vi "network-get_adapters.vi"(8 "error in (no error)":errorcluster) -> (0 "error out":errorcluster, 3 "adapter []":T1[](array[typedef]))   [LabVIEW 2015, in "lv-bin-windows.lvlib" / "v1.lvlib"]
uses:
  v1.lvlib
  _controls/adapter.ctl
  <userlib>/antonio-alexander/lv-bin/lv-bin/public/api/v1/v1.lvlib
panel:
  out "standard output":string
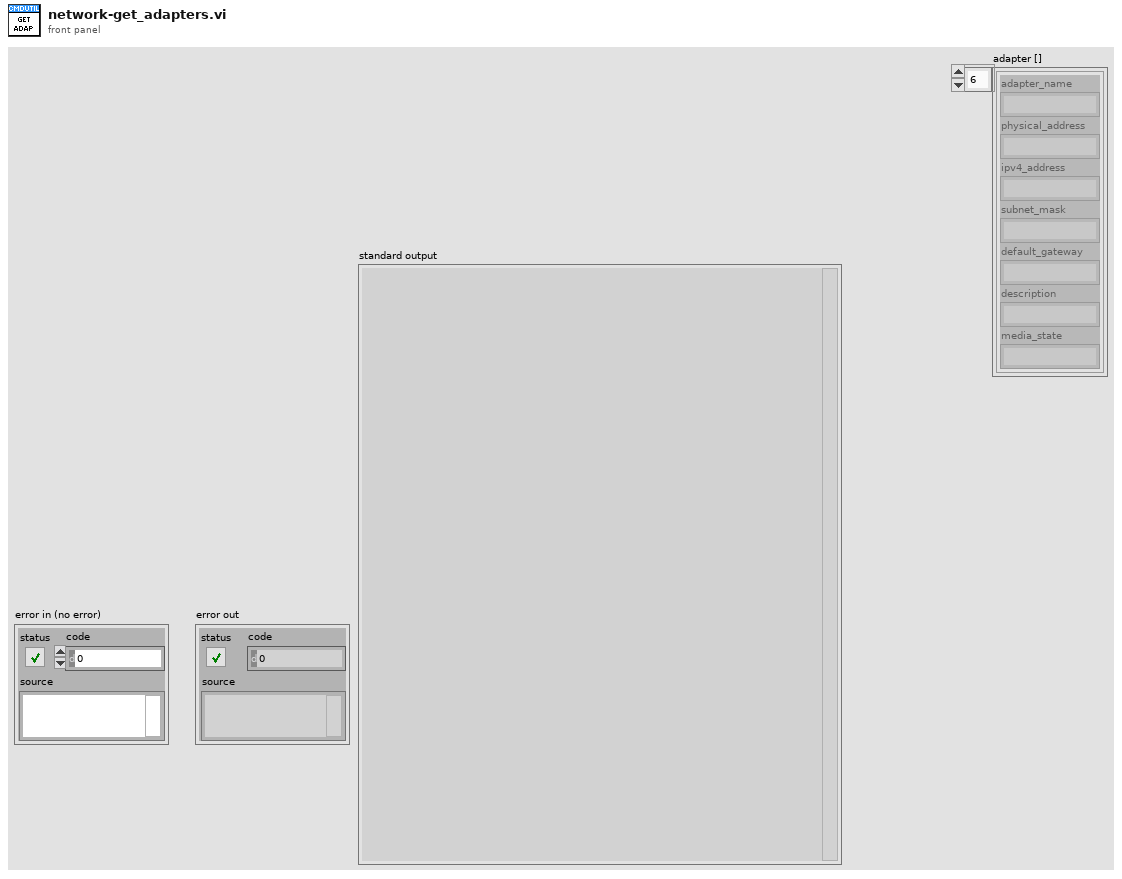
[diagram p1: front panel]
types:
  T1 = typedef "lv-bin-windows.lvlib/v1.lvlib/adapter.ctl" = cluster{"adapter_name":string, "physical_address":string, "ipv4_address":string, "subnet_mask":string, "default_gateway":string, "description":string, "media_state":string}
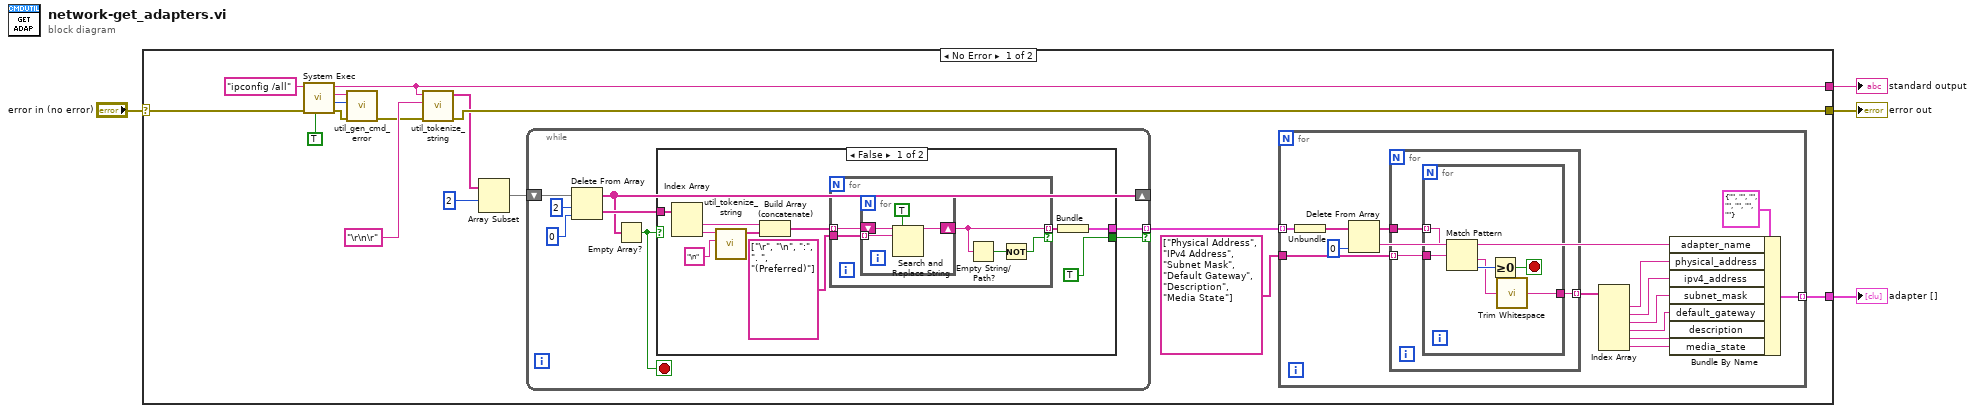
[diagram p0: block diagram]
diagram:
  n1 = case shown="No Error" "error in (no error)" {
    selector: "error in (no error)" -> [w18 w72]
    tunnel: [w11 _] -> w2
    tunnel: [w20 w72] -> w3
    tunnel: [w7 _] -> w1
    frame No Error {
      n2 = call <vilib>:"System Exec.vi"("run minimized? (F)"=TRUE, "error in (no error)"=w18, "command line"="ipconfig /all") -> ("error out"=w12:errorcluster, "return code"=w5:i32, "standard error"=w9:string, "standard output"=w11:string)  [unwired: 5 in]
      n3 = call <userlib>:"util_gen_cmd_error.vi"("error in (no error)"=w12, "return_code"=w5, "standard_error"=w9) -> ("error out"=w10:errorcluster)  [unwired: 8 in]
      n4 = call <userlib>:"util_tokenize_string.vi"("error in (no error)"=w10, "delimiter"="\r\n\r" ("delimiter ([\\s\\t\\n\\r]+)"), "input_string"=w11) -> ("error out"=w20:errorcluster, "before_match []"=w13:string[])  [unwired: 6 in, 1 out]
      n5 = Array Subset(array=w13, index=2 ("length")) -> (w16:string[])  [unwired: 1 in]
      n6 = while {
        shift-right: [w24] -> _
        shift-left: w16 -> [w28]
        tunnel: [w25] -> w8 mode=indexing if=w21
        stop <- w22 stop-if-true
        n7 = Delete From Array(array=w28, length=2, index=0) -> (deleted portion=w26:string[], array with subset deleted=w24:string[])
        n8 = Empty Array?(array=w24) -> (empty?=w22:bool)
        n9 = case shown="False" w22 {
          tunnel: w26 -> [w33 _]
          tunnel: [w35 _] -> w25
          tunnel: [TRUE _] -> w21
          frame False {
            n10 = Index Array(array=w33) -> (element #1=w31:string, element #2=w32:string)  [unwired: 2 in]
            n11 = call <userlib>:"util_tokenize_string.vi"("delimiter"="\n" ("delimiter ([\\s\\t\\n\\r]+)"), "input_string"=w32) -> ("before_match []"=w30:string[])  [unwired: 7 in, 2 out]
            n12 = Build Array (concatenate)(w31, w30) -> (w29:string[])
            n13 = for {
              tunnel: [w41] -> w36 mode=indexing if=w39
              tunnel: w29 -> [w43] mode=indexing
              tunnel: string[] ["\r", "\n", ":", ". ", "(Preferred)"] -> [w42]
              n14 = for {
                shift-right: [w46] -> w41
                shift-left: w43 -> [w47]
                tunnel: w42 -> [w44] mode=indexing
                n15 = Search and Replace String(replace all?=TRUE ("replace all? (F)"), input string=w47, search string=w44) -> (result string=w46:string)  [unwired: 5 in, 3 out]
              }
              n16 = Empty String/Path?(string/path=w41) -> (empty?=w40:bool)
              n17 = Not(x=w40) -> (.not. x?=w39:bool)
            }
            n18 = Bundle(w36) -> (w35:cluster{string[]})  [unwired: 1 in]
          }
          frame True {
          }
        }
      }
      n19 = for {
        tunnel: w8 -> [w62] mode=indexing
        tunnel: [w60] -> w7 mode=indexing
        tunnel: string[] ["Physical Address", "IPv4 Address", "Subnet Mask", "Default Gateway", "Description", "Media State"] -> [w56]
        n20 = Unbundle(w62) -> (w59:string[])
        n21 = Delete From Array(array=w59, index=0) -> (deleted portion=w55:string, array with subset deleted=w57:string[])  [unwired: 1 in]
        n22 = for {
          tunnel: w57 -> [w65]
          tunnel: w56 -> [w64] mode=indexing
          tunnel: [w63] -> w54 mode=indexing
          n23 = for {
            tunnel: w65 -> [w69] mode=indexing
            tunnel: w64 -> [w71]
            tunnel: [w67] -> w63
            stop <- w66 stop-if-true
            n24 = Match Pattern(string=w69, regular expression=w71) -> (after substring=w68:string, offset past match=w70:i32)  [unwired: 1 in, 2 out]
            n25 = Greater Or Equal To 0?(x=w70) -> (x >= 0?=w66:bool)
            n26 = call <vilib>:"Trim Whitespace.vi"("string"=w68) -> ("trimmed string"=w67:string)  [unwired: 1 in]
          }
        }
        n27 = Index Array(array=w54) -> (element #1=w53:string, element #2=w52:string, element #3=w51:string, element #4=w50:string, element #5=w49:string, element #6=w48:string)  [unwired: 6 in]
        n28 = Bundle By Name(cluster=T1 {"adapter_name"="", "physical_address"="", "ipv4_address"="", "subnet_mask"="", "default_gateway"="", "description"="", "media_state"=""} ("adapter"), "adapter_name"=w55, "physical_address"=w53, "ipv4_address"=w52, "subnet_mask"=w51, "default_gateway"=w50, "description"=w49, "media_state"=w48) -> (w60:T1)
      }
    }
    frame Error {
    }
  }
  "error out" <- w3
  "standard output" <- w2
  "adapter []" <- w1
